vi "Tree.vi"() -> ()   [LabVIEW 2019, in "xy_utilities.lvlib"]
uses:
  xy_utilities.lvlib
  User/User.lvclass
  subVIs/Append (double array).vi
  subVIs/Add float (multiple).vi
  subVIs/Subtract float (multiple).vi
  subVIs/Multiply float (multiple).vi
  subVIs/Divide float (multiple).vi
  subVIs/Add XY (multiple).vi
  subVIs/Subtract XY (multiple).vi
  subVIs/Multiply XY (multiple).vi
  subVIs/Divide XY (multiple).vi
  subVIs/Square Root (multiple).vi
  subVIs/Square (multiple).vi
  subVIs/Reciprocal (multiple).vi
  subVIs/Negate (multiple).vi
  subVIs/Log (multiple).vi
  subVIs/Add float (single).vi
  subVIs/Subtract float (single).vi
  subVIs/Multiply float (single).vi
  subVIs/Divide float (single).vi
  subVIs/Add XY (single).vi
  subVIs/Subtract XY (single).vi
  subVIs/Multiply XY (single).vi
  subVIs/Divide XY (single).vi
  subVIs/Square Root (single).vi
  subVIs/Square (single).vi
  subVIs/Reciprocal (single).vi
  subVIs/Negate (single).vi
  subVIs/Log (single).vi
  <vilib>/Analysis/6fits.llb/Remove Outliers (Range).vi
  <vilib>/Analysis/2dsp.llb/1D Auto Correlation (DBL).vi
  <vilib>/Analysis/2dsp.llb/Decimate (single shot, DBL).vi
  subVIs/Sort (multiple).vi
  subVIs/Reverse (multiple).vi
  subVIs/Decimate (multiple).vi
  subVIs/Subset (multiple).vi
  subVIs/Interpolate Y (multiple).vi
  subVIs/Append (multiple).vi
  subVIs/Split (multiple).vi
  subVIs/Remove Outliers (multiple).vi
  subVIs/Restrict X Range (multiple).vi
  subVIs/Sort (single).vi
  subVIs/Reverse (single).vi
  subVIs/Decimate (single).vi
  subVIs/Subset (single).vi
  subVIs/Interpolate Y (single).vi
  subVIs/Append (double scaler).vi
  subVIs/Append (single).vi
  subVIs/Split (single).vi
  subVIs/Remove Outliers (single).vi
  subVIs/Restrict X Range (single).vi
  subVIs/AutoCorrelation (single).vi
  subVIs/CrossCorrelation (single).vi
  subVIs/Swap X and Y (multiple).vi
  subVIs/Get X and Y (multiple).vi
  subVIs/XY to Waveform (multiple).vi
  subVIs/Get Size (multiple).vi
  subVIs/Max and Min (multiple).vi
  subVIs/Swap X and Y (single).vi
  subVIs/Get X and Y (single).vi
  subVIs/XY to Waveform (single).vi
  subVIs/Get Size (single).vi
  subVIs/Max and Min (single).vi
  <vilib>/Analysis/baseanly.llb/Mean (DBL).vi
  subVIs/Derivative (multiple).vi
  subVIs/Difference Quotient (multiple).vi
  subVIs/Linear Fit (multiple).vi
  subVIs/Interpolate (multiple).vi
  subVIs/Resample (multiple).vi
  subVIs/PS (multiple).vi
  subVIs/FFT (multiple).vi
  subVIs/Symmetrize (multiple).vi
  subVIs/Shift Zero (multiple).vi
  subVIs/Peak Detector (multiple).vi
  subVIs/Derivative (single).vi
  subVIs/Difference Quotient (single).vi
  subVIs/Linear Fit (single).vi
  subVIs/Interpolate (single).vi
  subVIs/Resample (single).vi
  subVIs/PS (single).vi
  subVIs/FFT (single).vi
  subVIs/Symmetrize (single).vi
  subVIs/Shift Zero (single).vi
  subVIs/Peak Detector (single).vi
  <vilib>/Analysis/3filter.llb/Savitzky-Golay Filter (DBL).vi
  subVIs/Zero Phase Lowpass Filter (multiple).vi
  subVIs/Moving Average (multiple).vi
  subVIs/Savitsky Golay Filter (multiple).vi
  subVIs/Savitsky Golay Weighted Filter (multiple).vi
  User/User (multiple).vi
  subVIs/Zero Phase Lowpass Filter (single).vi
  subVIs/Moving Average (single).vi
  subVIs/Savitsky Golay Filter (single).vi
  subVIs/Savitsky Golay Weighted Filter (single).vi
  User/User (single).vi
  subVIs/(x,y) to XY (multiple).vi
  subVIs/XY to (x,y) (multiple).vi
  subVIs/(x,y) to XY (single).vi
  subVIs/XY to (x,y) (single).vi
  subVIs/Waveform to XY (multiple).vi
  subVIs/Waveform to XY (single).vi
  <vilib>/Utility/error.llb/Clear Errors.vi
  Initialize.vi
  <vilib>/Analysis/6fits.llb/Linear Fit Intervals.vi
  <vilib>/Analysis/6fits.llb/Confidence Interval (Linear).vi
  <userlib>/_OpenG.lib/array/array.llb/Sort Array__ogtk.vi
  <userlib>/_OpenG.lib/array/array.llb/Sort 1D Array (DBL)__ogtk.vi
  <userlib>/_OpenG.lib/array/array.llb/Reorder Array2__ogtk.vi
  <userlib>/_OpenG.lib/array/array.llb/Reorder 1D Array2 (DBL)__ogtk.vi
  <vilib>/Utility/error.llb/Error Cluster From Error Code.vi
  <userlib>/_MGI/1D Array/MGI Threshold 1D Array Extended.vi
  <userlib>/_MGI/1D Array/MGI Interpolate 1D Array Extended.vi
  <vilib>/Waveform/WDTOps.llb/WDT Append Waveforms DBL.vi
  <vilib>/Analysis/2dsp.llb/1D Cross Correlation (DBL).vi
  <vilib>/measure/maresamp.llb/Resample Pair of Arrays (single shot).vi
  subVIs/Circular Buffer (waveform).vi
  subVIs/Circular Buffer (single).vi
  subVIs/Circular Buffer (waveforms).vi
  subVIs/Circular Buffer (multiple).vi
  subVIs/Circular Buffer (scaler).vi
  subVIs/Circular Buffer (array).vi
  <vilib>/Analysis/1siggen.llb/Ramp Pattern.vi
  <vilib>/Analysis/1siggen.llb/Ramp Pattern by Delta.vi
  <vilib>/gmath/interp.llb/Interpolate 1D.vi
  <vilib>/measure/maspectr.llb/FFT Power Spectrum and PSD for 1 Chan.vi
  <vilib>/measure/maspectr.llb/FFT Spectrum (Mag-Phase) for 1 Chan.vi
  <vilib>/measure/maresamp.llb/Resample Waveform (single shot).vi
  <vilib>/measure/maresamp.llb/Resample N Pairs of Arrays (single shot).vi
  <vilib>/Analysis/3filter.llb/FIR Windowed Coefficients.vi
  <vilib>/Analysis/3filter.llb/Zero Phase Filter (DBL).vi
  <vilib>/Waveform/WDTOps.llb/Waveform to XY Pairs.vi
  <vilib>/Waveform/WDTOps.llb/WDT Waveform to XY Pairs DBL.vi
  <vilib>/Analysis/NI_AALPro.lvlib
  <vilib>/Analysis/NI_AALBase.lvlib
  <vilib>/measure/NI_MAPro.lvlib
  <vilib>/ptbypt/NI_PtbyPt.lvlib
  <vilib>/Analysis/NI_AAL_SigProc.lvlib
panel:
  out "Array of XY-data":cluster{"X-array":dbl[], "Y-array":dbl[]}[](array[cluster])
  out "XY-data":cluster{"X-array":dbl[], "Y-array":dbl[]}
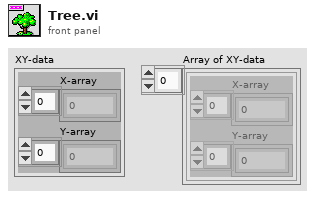
[diagram p1: front panel]
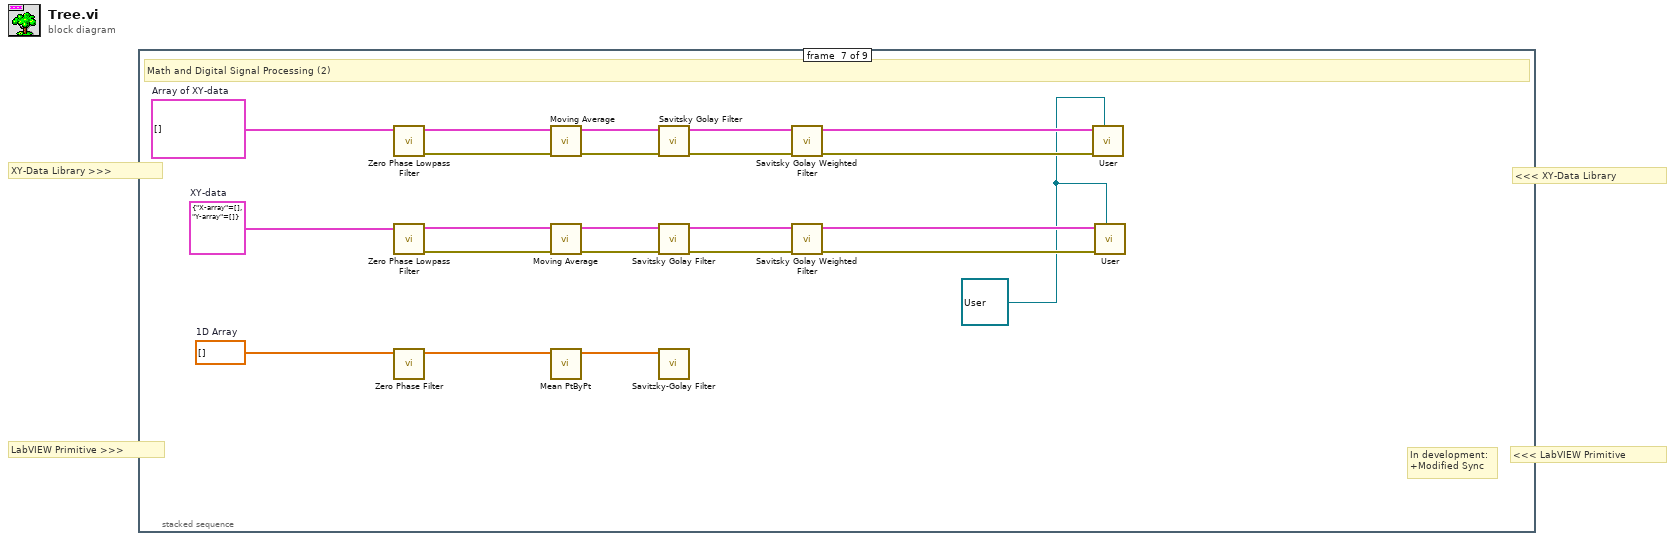
[diagram p0: block diagram]
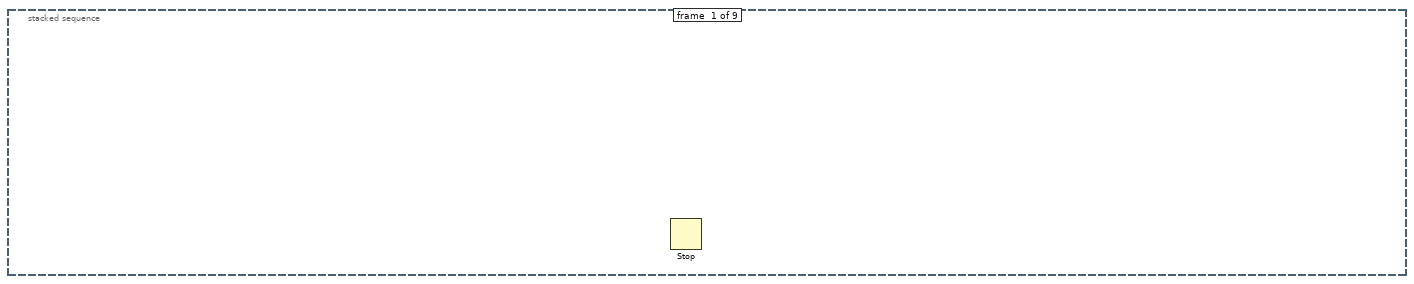
[diagram p2: hidden frame]
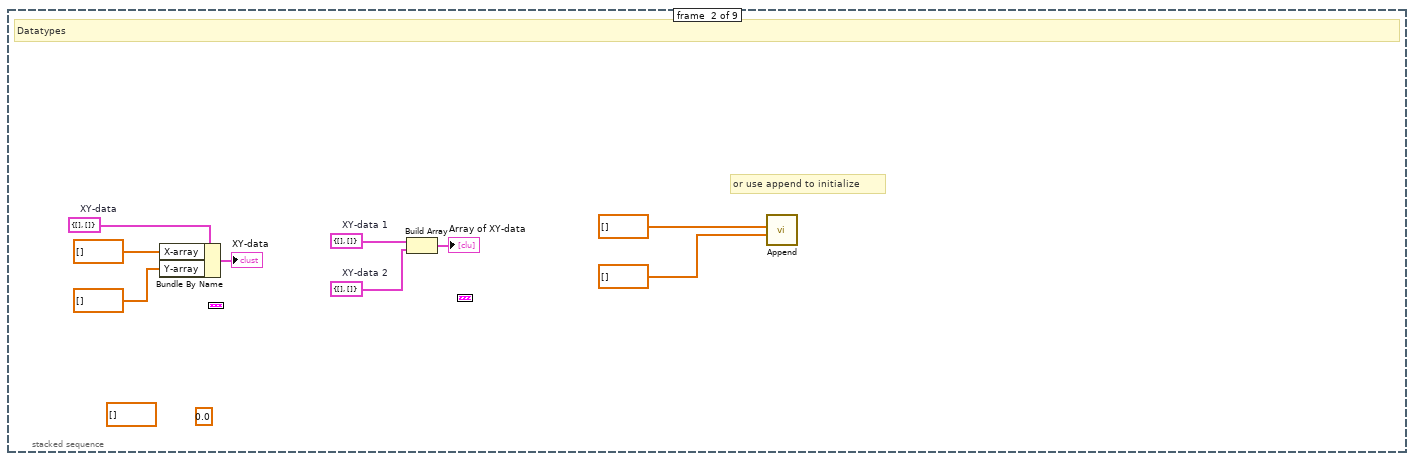
[diagram p3: hidden frame]
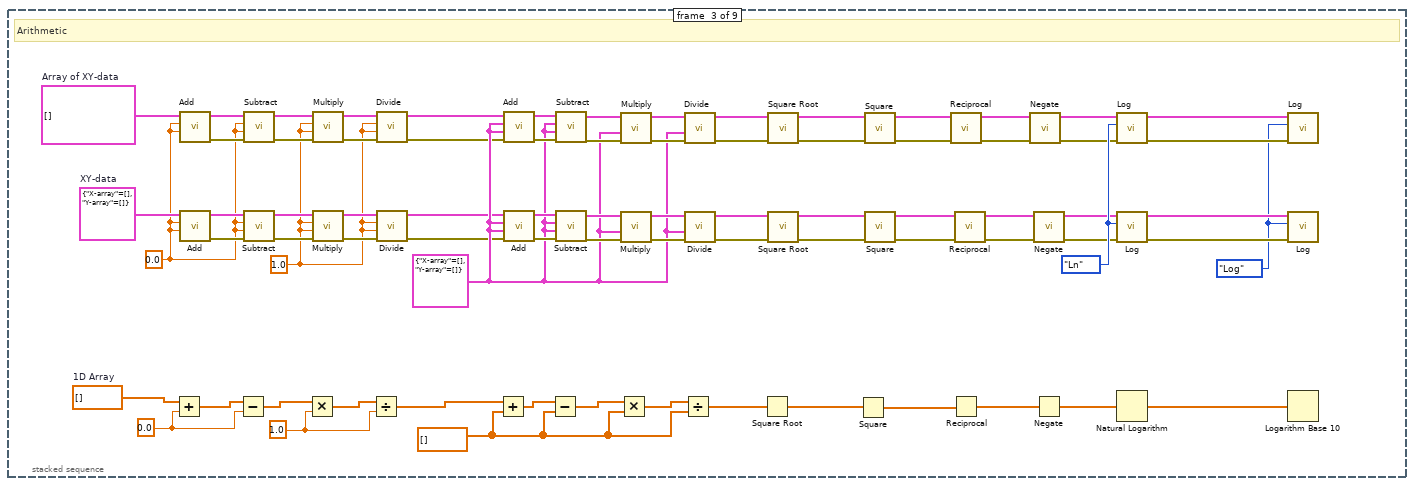
[diagram p4: hidden frame]
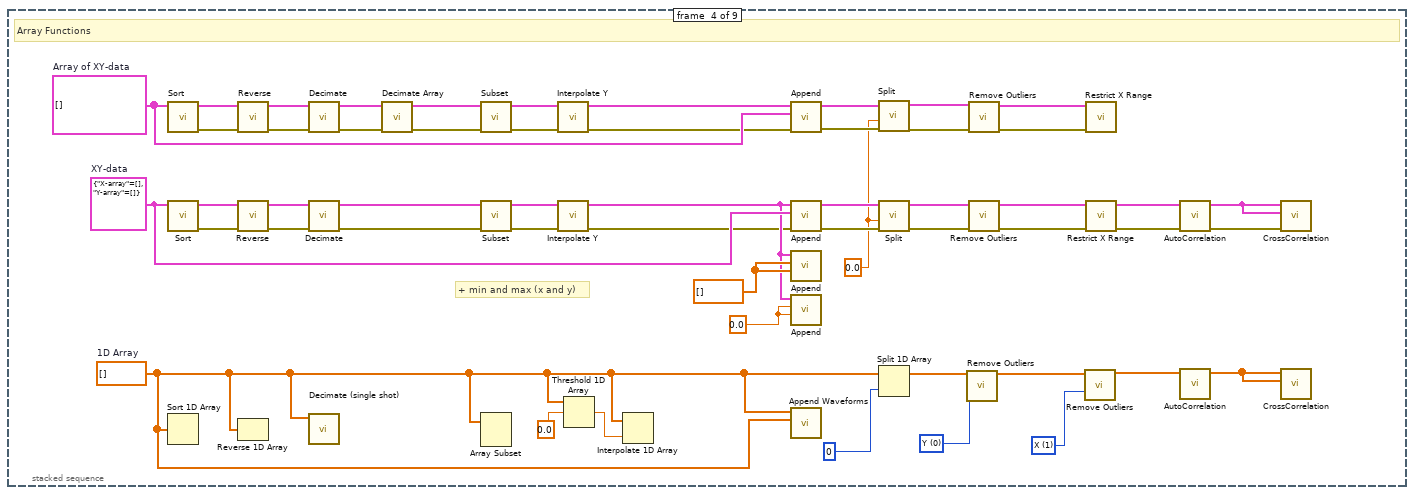
[diagram p5: hidden frame]
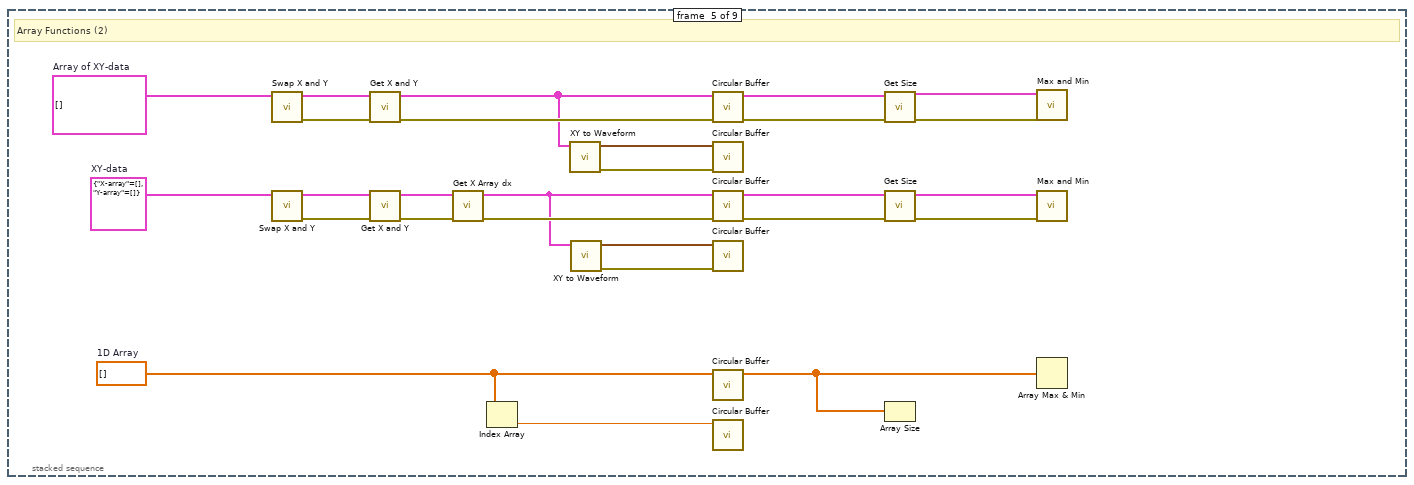
[diagram p6: hidden frame]
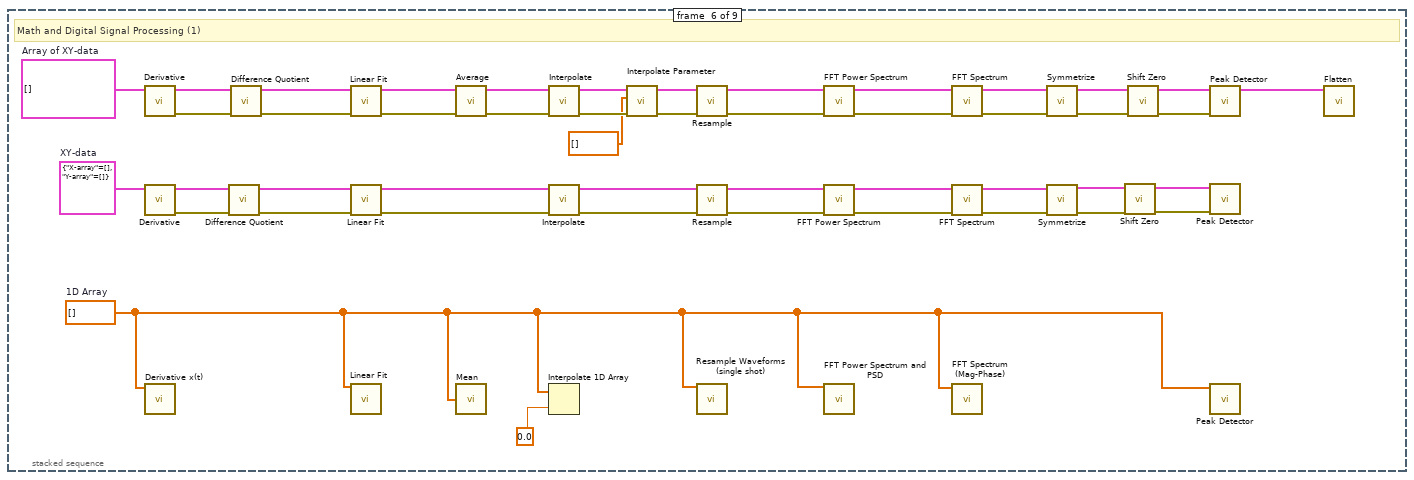
[diagram p7: hidden frame]
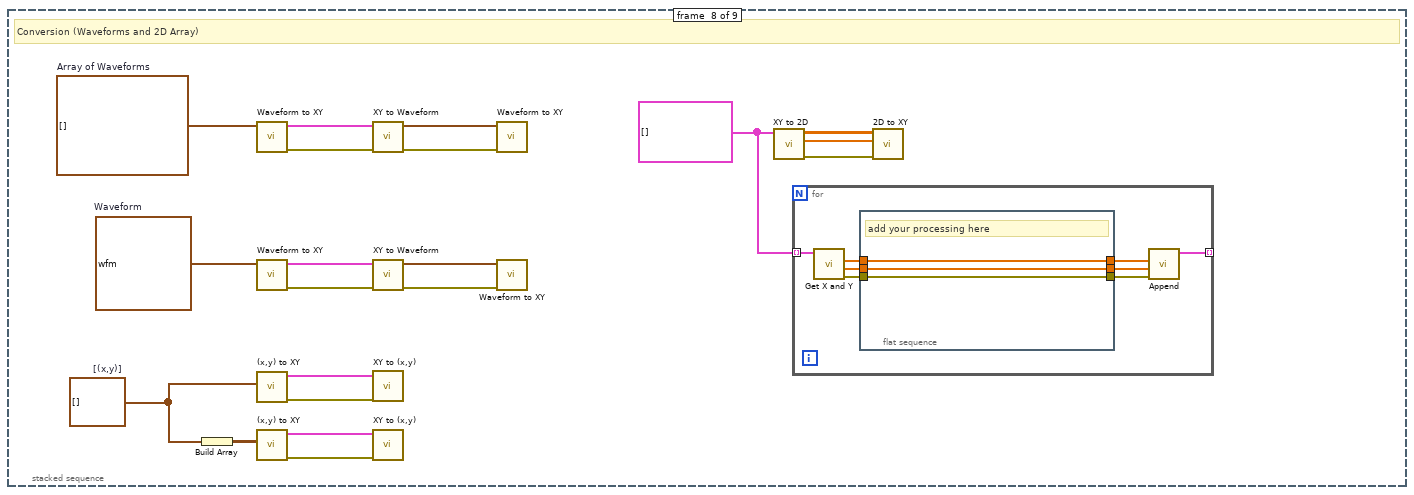
[diagram p8: hidden frame]
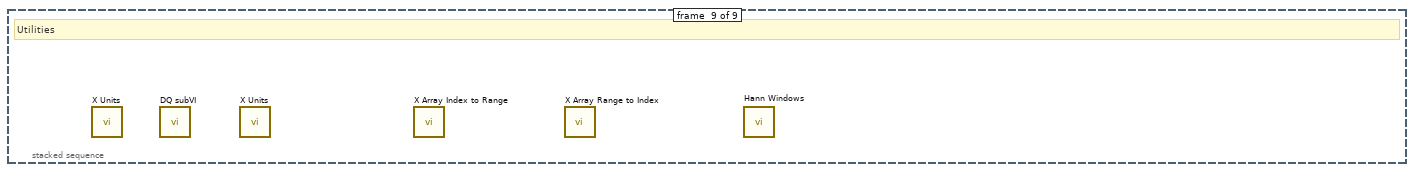
[diagram p9: hidden frame]
diagram:
  # "XY-Data Library >>>"
  # "LabVIEW Primitive >>>"
  # "<<< XY-Data Library"
  # "<<< LabVIEW Primitive"
  n1 = stacked-sequence {
    frame #0 {
      n2 = Stop() -> ()  [unwired: 1 in]
    }
    frame #1 {
      (unwired) 0.0
      (unwired) dbl[] [] ("Y-array")
      w7 = cluster{"X-array":dbl[], "Y-array":dbl[]} {"X-array"=[], "Y-array"=[]}  # XY-data 2
      w8 = cluster{"X-array":dbl[], "Y-array":dbl[]} {"X-array"=[], "Y-array"=[]}  # XY-data 1
      w6 = cluster{"X-array":dbl[], "Y-array":dbl[]} {"X-array"=[], "Y-array"=[]}  # XY-data
      # "or use append to initialize"
      # "Datatypes"
      n3 = Bundle By Name(cluster=w6, "X-array"=dbl[] [], "Y-array"=dbl[] []) -> (→"XY-data":cluster{"X-array":dbl[], "Y-array":dbl[]})
      n4 = Build Array(w8, w7) -> (→"Array of XY-data":cluster{"X-array":dbl[], "Y-array":dbl[]}[])
      n5 = call-poly "Append.vi"("Y-array"=dbl[] [], "X-array"=dbl[] []) -> ()  [unwired: 8 in, 2 out]
    }
    frame #2 {
      w35 = enum16{"Ln", "Log"}."Log" ("Type")
      w41 = enum16{"Ln", "Log"}."Ln" ("Type")
      w51 = cluster{"X-array":dbl[], "Y-array":dbl[]} {"X-array"=[], "Y-array"=[]} ("XY-data in")
      w60 = 1.0 ("x (0)")
      w69 = 0.0 ("x (0)")
      w48 = dbl[] []
      w62 = 1.0 ("x (0)")
      w63 = 0.0 ("x (0)")
      w42 = dbl[] []  # 1D Array
      w85 = cluster{"X-array":dbl[], "Y-array":dbl[]}[] []  # Array of XY-data
      w84 = cluster{"X-array":dbl[], "Y-array":dbl[]} {"X-array"=[], "Y-array"=[]}  # XY-data
      # "Arithmetic"
      n6 = Add(x=w42, y=w63) -> (x+y=w83:dbl[])
      n7 = call-poly "Add.vi"("y (0)"=w69, "x (0)"=w69, "XY-data"=w85) -> ("error out"=w74:errorcluster, "XY-data out"=w75:cluster{"X-array":dbl[], "Y-array":dbl[]}[])  [unwired: 7 in]
      n8 = call-poly "Add.vi"("y (0)"=w69, "x (0)"=w69, "XY-data"=w84) -> ("error out"=w70:errorcluster, "XY-data out"=w71:cluster{"X-array":dbl[], "Y-array":dbl[]})  [unwired: 7 in]
      n9 = Subtract(x=w83, y=w63) -> (x-y=w82:dbl[])
      n10 = call-poly "Subtract.vi"("error in (no error)"=w74, "y (0)"=w69, "x (0)"=w69, "XY-data"=w75) -> ("error out"=w72:errorcluster, "XY-data out"=w73:cluster{"X-array":dbl[], "Y-array":dbl[]}[])  [unwired: 6 in]
      n11 = call-poly "Subtract.vi"("error in (no error)"=w70, "y (0)"=w69, "x (0)"=w69, "XY-data"=w71) -> ("error out"=w77:errorcluster, "XY-data out"=w78:cluster{"X-array":dbl[], "Y-array":dbl[]})  [unwired: 6 in]
      n12 = Multiply(x=w82, y=w62) -> (x*y=w64:dbl[])
      n13 = call-poly "Multiply.vi"("error in (no error)"=w72, "y (1)"=w60, "x (1)"=w60, "XY-data"=w73) -> ("error out"=w79:errorcluster, "XY-data out"=w81:cluster{"X-array":dbl[], "Y-array":dbl[]}[])  [unwired: 6 in]
      n14 = call-poly "Multiply.vi"("error in (no error)"=w77, "y (1)"=w60, "x (1)"=w60, "XY-data"=w78) -> ("error out"=w76:errorcluster, "XY-data out"=w80:cluster{"X-array":dbl[], "Y-array":dbl[]})  [unwired: 6 in]
      n15 = Divide(x=w64, y=w62) -> (x/y=w43:dbl[])
      n16 = call-poly "Divide.vi"("error in (no error)"=w79, "y (1)"=w60, "x (1)"=w60, "XY-data"=w81) -> ("error out"=w46:errorcluster, "XY-data out"=w47:cluster{"X-array":dbl[], "Y-array":dbl[]}[])  [unwired: 6 in]
      n17 = call-poly "Divide.vi"("error in (no error)"=w76, "y (1)"=w60, "x (1)"=w60, "XY-data"=w80) -> ("error out"=w44:errorcluster, "XY-data out"=w45:cluster{"X-array":dbl[], "Y-array":dbl[]})  [unwired: 6 in]
      n18 = Add(x=w43, y=w48) -> (x+y=w61:dbl[])
      n19 = call-poly "Add.vi"("error in (no error)"=w46, "y"=w51, "x"=w51, "XY-data"=w47) -> ("error out"=w67:errorcluster, "XY-data out"=w66:cluster{"X-array":dbl[], "Y-array":dbl[]}[])  [unwired: 6 in]
      n20 = call-poly "Add.vi"("error in (no error)"=w44, "y"=w51, "x"=w51, "XY-data"=w45) -> ("error out"=w65:errorcluster, "XY-data out"=w68:cluster{"X-array":dbl[], "Y-array":dbl[]})  [unwired: 6 in]
      n21 = Subtract(x=w61, y=w48) -> (x-y=w49:dbl[])
      n22 = call-poly "Subtract.vi"("error in (no error)"=w67, "y"=w51, "x"=w51, "XY-data"=w66) -> ("error out"=w54:errorcluster, "XY-data out"=w55:cluster{"X-array":dbl[], "Y-array":dbl[]}[])  [unwired: 6 in]
      n23 = call-poly "Subtract.vi"("error in (no error)"=w65, "y"=w51, "x"=w51, "XY-data"=w68) -> ("error out"=w52:errorcluster, "XY-data out"=w53:cluster{"X-array":dbl[], "Y-array":dbl[]})  [unwired: 6 in]
      n24 = Multiply(x=w49, y=w48) -> (x*y=w50:dbl[])
      n25 = call-poly "Multiply.vi"("error in (no error)"=w54, "y"=w51, "XY-data"=w55) -> ("error out"=w58:errorcluster, "XY-data out"=w56:cluster{"X-array":dbl[], "Y-array":dbl[]}[])  [unwired: 7 in]
      n26 = call-poly "Multiply.vi"("error in (no error)"=w52, "y"=w51, "XY-data"=w53) -> ("error out"=w59:errorcluster, "XY-data out"=w57:cluster{"X-array":dbl[], "Y-array":dbl[]})  [unwired: 7 in]
      n27 = Divide(x=w50, y=w48) -> (x/y=w33:dbl[])
      n28 = call-poly "Divide.vi"("error in (no error)"=w58, "y"=w51, "XY-data"=w56) -> ("error out"=w28:errorcluster, "XY-data out"=w29:cluster{"X-array":dbl[], "Y-array":dbl[]}[])  [unwired: 7 in]
      n29 = call-poly "Divide.vi"("error in (no error)"=w59, "y"=w51, "XY-data"=w57) -> ("error out"=w18:errorcluster, "XY-data out"=w19:cluster{"X-array":dbl[], "Y-array":dbl[]})  [unwired: 7 in]
      n30 = Square Root(x=w33) -> (sqrt(x)=w32:dbl[])
      n31 = call-poly "Square Root.vi"("error in (no error)"=w28, "XY-data"=w29) -> ("error out"=w26:errorcluster, "XY-data out"=w27:cluster{"X-array":dbl[], "Y-array":dbl[]}[])  [unwired: 8 in]
      n32 = call-poly "Square Root.vi"("error in (no error)"=w18, "XY-data"=w19) -> ("error out"=w16:errorcluster, "XY-data out"=w17:cluster{"X-array":dbl[], "Y-array":dbl[]})  [unwired: 8 in]
      n33 = Square(x=w32) -> (x^2=w31:dbl[])
      n34 = call-poly "Square.vi"("error in (no error)"=w26, "XY-data"=w27) -> ("error out"=w24:errorcluster, "XY-data out"=w25:cluster{"X-array":dbl[], "Y-array":dbl[]}[])  [unwired: 8 in]
      n35 = call-poly "Square.vi"("error in (no error)"=w16, "XY-data"=w17) -> ("error out"=w14:errorcluster, "XY-data out"=w15:cluster{"X-array":dbl[], "Y-array":dbl[]})  [unwired: 8 in]
      n36 = call-poly "Reciprocal.vi"("error in (no error)"=w24, "XY-data"=w25) -> ("error out"=w22:errorcluster, "XY-data out"=w23:cluster{"X-array":dbl[], "Y-array":dbl[]}[])  [unwired: 8 in]
      n37 = Reciprocal(x=w31) -> (1/x=w36:dbl[])
      n38 = call-poly "Reciprocal.vi"("error in (no error)"=w14, "XY-data"=w15) -> ("error out"=w12:errorcluster, "XY-data out"=w13:cluster{"X-array":dbl[], "Y-array":dbl[]})  [unwired: 8 in]
      n39 = call-poly "Negate.vi"("error in (no error)"=w22, "XY-data"=w23) -> ("error out"=w20:errorcluster, "XY-data out"=w21:cluster{"X-array":dbl[], "Y-array":dbl[]}[])  [unwired: 8 in]
      n40 = call-poly "Negate.vi"("error in (no error)"=w12, "XY-data"=w13) -> ("error out"=w10:errorcluster, "XY-data out"=w11:cluster{"X-array":dbl[], "Y-array":dbl[]})  [unwired: 8 in]
      n41 = Negate(x=w36) -> (-x=w30:dbl[])
      n42 = call-poly "Log.vi"("error in (no error)"=w20, "Type"=w41, "XY-data"=w21) -> ("error out"=w39:errorcluster, "XY-data out"=w40:cluster{"X-array":dbl[], "Y-array":dbl[]}[])  [unwired: 7 in]
      n43 = call-poly "Log.vi"("error in (no error)"=w10, "Type"=w41, "XY-data"=w11) -> ("error out"=w37:errorcluster, "XY-data out"=w38:cluster{"X-array":dbl[], "Y-array":dbl[]})  [unwired: 7 in]
      n44 = Natural Logarithm(1:w30) -> (0:w34:dbl[])
      n45 = call-poly "Log.vi"("error in (no error)"=w39, "Type"=w35, "XY-data"=w40) -> ()  [unwired: 7 in, 2 out]
      n46 = call-poly "Log.vi"("error in (no error)"=w37, "Type"=w35, "XY-data"=w38) -> ()  [unwired: 7 in, 2 out]
      n47 = Logarithm Base 10(1:w34) -> ()  [unwired: 1 out]
    }
    frame #3 {
      w92 = 0.0 ("index")
      w112 = dbl[] [] ("1D Array")
      w113 = u16 1 items=["Y", "X", "X and Y"] ("range type")
      w114 = u16 0 items=["Y", "X", "X and Y"] ("range type")
      w111 = 0.0 ("threshold y")
      w98 = dbl[] []  # 1D Array
      w109 = cluster{"X-array":dbl[], "Y-array":dbl[]}[] []  # Array of XY-data
      w110 = cluster{"X-array":dbl[], "Y-array":dbl[]} {"X-array"=[], "Y-array"=[]}  # XY-data
      # "+ min and max (x and y)"
      # "Array Functions"
      n48 = call-poly "Sort.vi"("XY-data"=w109) -> ("error out"=w133:errorcluster, "Sorted XY-data out"=w134:cluster{"X-array":dbl[], "Y-array":dbl[]}[])  [unwired: 8 in, 1 out]
      n49 = call-poly "Sort.vi"("XY-data"=w110) -> ("error out"=w129:errorcluster, "Sorted XY-data out"=w130:cluster{"X-array":dbl[], "Y-array":dbl[]})  [unwired: 8 in, 1 out]
      n50 = Sort 1D Array(array=w98) -> ()  [unwired: 1 out]
      n51 = call-poly "Reverse.vi"("error in (no error)"=w133, "XY-data"=w134) -> ("error out"=w131:errorcluster, "Reversed XY-data out"=w132:cluster{"X-array":dbl[], "Y-array":dbl[]}[])  [unwired: 8 in]
      n52 = call-poly "Reverse.vi"("error in (no error)"=w129, "XY-data"=w130) -> ("error out"=w136:errorcluster, "Reversed XY-data out"=w135:cluster{"X-array":dbl[], "Y-array":dbl[]})  [unwired: 8 in]
      n53 = Reverse 1D Array(array=w98) -> ()  [unwired: 1 out]
      n54 = call-poly "Decimate.vi"("error in (no error)"=w131, "XY-data"=w132) -> ("error out"=w128:errorcluster, "Decimated XY-data out"=w127:cluster{"X-array":dbl[], "Y-array":dbl[]}[])  [unwired: 8 in]
      n55 = call-poly "Decimate.vi"("error in (no error)"=w136, "XY-data"=w135) -> ("error out"=w137:errorcluster, "Decimated XY-data out"=w138:cluster{"X-array":dbl[], "Y-array":dbl[]})  [unwired: 8 in]
      n56 = call-poly <vilib>:"Decimate (single shot).vi"("X"=w98) -> ()  [unwired: 9 in, 2 out]
      n57 = call "Decimate Array.vi"("error in (no error)"=w128, "XY-data"=w127) -> ("error out"=w126:errorcluster, "Decimated XY-data out"=w125:cluster{"X-array":dbl[], "Y-array":dbl[]}[])  [unwired: 8 in]
      n58 = call-poly "Subset.vi"("error in (no error)"=w126, "XY-data"=w125) -> ("error out"=w123:errorcluster, "Subset XY-data out"=w124:cluster{"X-array":dbl[], "Y-array":dbl[]}[])  [unwired: 8 in]
      n59 = call-poly "Subset.vi"("error in (no error)"=w137, "XY-data"=w138) -> ("error out"=w121:errorcluster, "XY-data out"=w122:cluster{"X-array":dbl[], "Y-array":dbl[]})  [unwired: 8 in]
      n60 = Array Subset "Array Subset"(array=w98) -> ()  [unwired: 2 in, 1 out]
      n61 = call-poly "Interpolate Y.vi"("error in (no error)"=w123, "XY-data"=w124) -> ("error out"=w106:errorcluster, "XY-data out"=w107:cluster{"X-array":dbl[], "Y-array":dbl[]}[])  [unwired: 7 in, 1 out]
      n62 = call-poly "Interpolate Y.vi"("error in (no error)"=w121, "XY-data"=w122) -> ("error out"=w104:errorcluster, "XY-data out"=w105:cluster{"X-array":dbl[], "Y-array":dbl[]})  [unwired: 7 in, 1 out]
      n63 = Threshold 1D Array(2:0.0 ("threshold y"), 3:w98) -> (0:w120:dbl)  [unwired: 1 in]
      n64 = Interpolate 1D Array(1:w120, 2:w98) -> ()  [unwired: 1 out]
      n65 = call-poly "Append.vi"("error in (no error)"=w106, "XY-data (B)"=w109, "XY-data (A)"=w107) -> ("error out"=w102:errorcluster, "XY-data out"=w103:cluster{"X-array":dbl[], "Y-array":dbl[]}[])  [unwired: 7 in]
      n66 = call-poly "Append.vi"("error in (no error)"=w104, "XY-data (B)"=w110, "XY-data (A)"=w105) -> ("error out"=w95:errorcluster, "XY-data out"=w100:cluster{"X-array":dbl[], "Y-array":dbl[]})  [unwired: 7 in]
      n67 = call-poly "Append.vi"("Y-array"=w112, "X-array"=w112, "XY-data (A)"=w105) -> ()  [unwired: 7 in, 2 out]
      n68 = call-poly "Append.vi"("Y"=w111, "X"=w111, "XY-data (A)"=w105) -> ()  [unwired: 7 in, 2 out]
      n69 = call-poly <vilib>:"Append Waveforms.vi"("waveform B"=w98, "waveform A"=w98) -> ()  [unwired: 8 in, 2 out]
      n70 = call-poly "Split.vi"("error in (no error)"=w102, "fractional index"=w92, "XY-data"=w103) -> ("error out"=w96:errorcluster, "XY-data (A) out"=w101:cluster{"X-array":dbl[], "Y-array":dbl[]}[])  [unwired: 6 in, 1 out]
      n71 = call-poly "Split.vi"("error in (no error)"=w95, "fractional index"=w92, "XY-data"=w100) -> ("error out"=w94:errorcluster, "XY-data (A) out"=w99:cluster{"X-array":dbl[], "Y-array":dbl[]})  [unwired: 6 in, 1 out]
      n72 = Split 1D Array(array=w98, index=0) -> (first subarray=w97:dbl[])  [unwired: 1 out]
      n73 = call-poly <vilib>:"Remove Outliers.vi"("Y"=w97, "range type"=w114) -> ("Y Out"=w115:dbl[])  [unwired: 9 in, 4 out]
      n74 = call-poly <vilib>:"Remove Outliers.vi"("error in (no error)"=w96, "XY-data"=w101) -> ("error out"=w118:errorcluster, "XY-data out"=w119:cluster{"X-array":dbl[], "Y-array":dbl[]}[])  [unwired: 8 in]
      n75 = call-poly <vilib>:"Remove Outliers.vi"("error in (no error)"=w94, "XY-data"=w99) -> ("error out"=w117:errorcluster, "XY-data out"=w116:cluster{"X-array":dbl[], "Y-array":dbl[]})  [unwired: 8 in]
      n76 = call-poly <vilib>:"Remove Outliers.vi"("Y"=w115, "range type"=w113) -> ("Y Out"=w87:dbl[])  [unwired: 9 in, 4 out]
      n77 = call-poly "Restrict X Range.vi"("error in (no error)"=w118, "XY-data"=w119) -> ()  [unwired: 8 in, 2 out]
      n78 = call-poly "Restrict X Range.vi"("error in (no error)"=w117, "XY-data"=w116) -> ("error out"=w90:errorcluster, "XY-data out"=w91:cluster{"X-array":dbl[], "Y-array":dbl[]})  [unwired: 8 in]
      n79 = call-poly <vilib>:"AutoCorrelation.vi"("error in (no error)"=w90, "XY-data a"=w91) -> ("error out"=w89:errorcluster, "XY-data a out"=w88:cluster{"X-array":dbl[], "Y-array":dbl[]})  [unwired: 8 in]
      n80 = call-poly <vilib>:"AutoCorrelation.vi"("X"=w87) -> ("Rxx"=w86:dbl[])  [unwired: 9 in, 1 out]
      n81 = call-poly <vilib>:"CrossCorrelation.vi"("error in (no error)"=w89, "XY-data b"=w88, "XY-data a"=w88) -> ()  [unwired: 6 in, 3 out]
      n82 = call-poly <vilib>:"CrossCorrelation.vi"("Y"=w86, "X"=w86) -> ()  [unwired: 8 in, 2 out]
    }
    frame #4 {
      w151 = dbl[] []  # 1D Array
      w162 = cluster{"X-array":dbl[], "Y-array":dbl[]}[] []  # Array of XY-data
      w160 = cluster{"X-array":dbl[], "Y-array":dbl[]} {"X-array"=[], "Y-array"=[]}  # XY-data
      # "Array Functions (2)"
      n83 = call-poly "Swap X and Y.vi"("XY-data"=w162) -> ("error out"=w165:errorcluster, "XY-data out"=w161:cluster{"X-array":dbl[], "Y-array":dbl[]}[])  [unwired: 9 in]
      n84 = call-poly "Swap X and Y.vi"("XY-data"=w160) -> ("error out"=w163:errorcluster, "XY-data out"=w164:cluster{"X-array":dbl[], "Y-array":dbl[]})  [unwired: 9 in]
      n85 = call-poly "Get X and Y.vi"("error in (no error)"=w165, "XY-data"=w161) -> ("error out"=w158:errorcluster, "XY-data out"=w149:cluster{"X-array":dbl[], "Y-array":dbl[]}[])  [unwired: 6 in, 2 out]
      n86 = call-poly "Get X and Y.vi"("error in (no error)"=w163, "XY-data"=w164) -> ("error out"=w156:errorcluster, "XY-data out"=w159:cluster{"X-array":dbl[], "Y-array":dbl[]})  [unwired: 6 in, 2 out]
      n87 = call "Get X Array dx.vi"("error in (no error)"=w156, "XY-data"=w159) -> ("error out"=w157:errorcluster, "XY-data out"=w148:cluster{"X-array":dbl[], "Y-array":dbl[]})  [unwired: 6 in, 2 out]
      n88 = Index Array(array=w151) -> (element=w150:dbl)  [unwired: 1 in]
      n89 = call-poly "XY to Waveform.vi"("XY-data in"=w149) -> ("error out"=w145:errorcluster, "Waveform out"=w146:waveform(dbl)[])  [unwired: 8 in, 1 out]
      n90 = call-poly "XY to Waveform.vi"("XY-data in"=w148) -> ("error out"=w144:errorcluster, "Waveform out"=w147:waveform(dbl))  [unwired: 8 in, 1 out]
      n91 = call-poly "Circular Buffer.vi"("error in"=w158, "XY-data"=w149) -> ("error out"=w152:errorcluster, "XY-data out"=w154:cluster{"X-array":dbl[], "Y-array":dbl[]}[])  [unwired: 8 in]
      n92 = call-poly "Circular Buffer.vi"("error in"=w145, "Waveform in"=w146) -> ()  [unwired: 8 in, 2 out]
      n93 = call-poly "Circular Buffer.vi"("error in"=w157, "XY-data"=w148) -> ("error out"=w153:errorcluster, "XY-data out"=w155:cluster{"X-array":dbl[], "Y-array":dbl[]})  [unwired: 8 in]
      n94 = call-poly "Circular Buffer.vi"("error in"=w144, "Waveform in"=w147) -> ()  [unwired: 8 in, 2 out]
      n95 = call-poly "Circular Buffer.vi"("Array in"=w151) -> ("Array out"=w139:dbl[])  [unwired: 9 in, 1 out]
      n96 = call-poly "Circular Buffer.vi"("Element in"=w150) -> ()  [unwired: 9 in, 2 out]
      n97 = call-poly "Get Size.vi"("error in (no error)"=w152, "XY-data"=w154) -> ("error out"=w143:errorcluster, "XY-data out"=w142:cluster{"X-array":dbl[], "Y-array":dbl[]}[])  [unwired: 6 in, 2 out]
      n98 = call-poly "Get Size.vi"("error in (no error)"=w153, "XY-data"=w155) -> ("error out"=w140:errorcluster, "XY-data out"=w141:cluster{"X-array":dbl[], "Y-array":dbl[]})  [unwired: 6 in, 2 out]
      n99 = Array Size(array=w139) -> ()  [unwired: 1 out]
      n100 = call-poly "Max and Min.vi"("error in (no error)"=w143, "XY-data"=w142) -> ()  [unwired: 6 in, 4 out]
      n101 = call-poly "Max and Min.vi"("error in (no error)"=w140, "XY-data"=w141) -> ()  [unwired: 6 in, 4 out]
      n102 = Array Max & Min(array=w139) -> ()  [unwired: 4 out]
    }
    frame #5 {
      w169 = dbl[] []  # 1D Array
      w200 = cluster{"X-array":dbl[], "Y-array":dbl[]}[] []  # Array of XY-data
      w199 = cluster{"X-array":dbl[], "Y-array":dbl[]} {"X-array"=[], "Y-array"=[]}  # XY-data
      # "Math and Digital Signal Processing (1)"
      n103 = call-poly "Derivative.vi"("XY-data"=w200) -> ("error out"=w182:errorcluster, "XY-data out"=w183:cluster{"X-array":dbl[], "Y-array":dbl[]}[])  [unwired: 8 in, 1 out]
      n104 = call-poly "Derivative.vi"("XY-data"=w199) -> ("error out"=w172:errorcluster, "XY-data out"=w176:cluster{"X-array":dbl[], "Y-array":dbl[]})  [unwired: 8 in, 1 out]
      n105 = call <vilib>:"Derivative x(t).vi"("X"=w169) -> ()  [unwired: 9 in, 2 out]
      n106 = call-poly "Difference Quotient.vi"("error in (no error)"=w172, "XY-data"=w176) -> ("error out"=w177:errorcluster, "XY-data out"=w175:cluster{"X-array":dbl[], "Y-array":dbl[]})  [unwired: 7 in, 1 out]
      n107 = call-poly "Difference Quotient.vi"("error in (no error)"=w182, "XY-data"=w183) -> ("error out"=w180:errorcluster, "XY-data out"=w181:cluster{"X-array":dbl[], "Y-array":dbl[]}[])  [unwired: 7 in, 1 out]
      n108 = call-poly <vilib>:"Linear Fit.vi"("error in (no error)"=w180, "XY-data"=w181) -> ("error out"=w179:errorcluster, "XY-data out"=w178:cluster{"X-array":dbl[], "Y-array":dbl[]}[])  [unwired: 3 in, 5 out]
      n109 = call-poly <vilib>:"Linear Fit.vi"("error in (no error)"=w177, "XY-data"=w175) -> ("error out"=w173:errorcluster, "XY-data out"=w174:cluster{"X-array":dbl[], "Y-array":dbl[]})  [unwired: 3 in, 5 out]
      n110 = call <vilib>:"Linear Fit.vi"("Y"=w169) -> ()  [unwired: 10 in, 5 out]
      n111 = call "Average.vi"("error in (no error)"=w179, "XY-data"=w178) -> ("error out"=w205:errorcluster, "XY-data out"=w206:cluster{"X-array":dbl[], "Y-array":dbl[]}[])  [unwired: 7 in, 1 out]
      n112 = call-poly <vilib>:"Mean.vi"("X"=w169) -> ()  [unwired: 2 out]
      n113 = call-poly "Interpolate.vi"("error in (no error)"=w205, "XY-data"=w206) -> ("error out"=w187:errorcluster, "Interpolated XY-data out"=w189:cluster{"X-array":dbl[], "Y-array":dbl[]}[])  [unwired: 8 in]
      n114 = call-poly "Interpolate.vi"("error in (no error)"=w173, "XY-data"=w174) -> ("error out"=w207:errorcluster, "Interpolated XY-data out"=w190:cluster{"X-array":dbl[], "Y-array":dbl[]})  [unwired: 8 in]
      n115 = Interpolate 1D Array(1:0.0 ("fractional index or x"), 2:w169) -> ()  [unwired: 1 out]
      n116 = call "Interpolate Parameter.vi"("error in (no error)"=w187, "Parameter-array"=dbl[] [] ("1D Array"), "XY-data"=w189) -> ("error out"=w186:errorcluster, "Interpolated XY-data out"=w188:cluster{"X-array":dbl[], "Y-array":dbl[]}[])  [unwired: 6 in, 1 out]
      n117 = call-poly "Resample.vi"("error in (no error)"=w186, "XY-data"=w188) -> ("error out"=w203:errorcluster, "Resampled XY-data out"=w204:cluster{"X-array":dbl[], "Y-array":dbl[]}[])  [unwired: 8 in]
      n118 = call-poly "Resample.vi"("error in (no error)"=w207, "XY-data"=w190) -> ("error out"=w201:errorcluster, "Resampled XY-data out"=w202:cluster{"X-array":dbl[], "Y-array":dbl[]})  [unwired: 8 in]
      n119 = call-poly <vilib>:"Resample Waveforms (single shot).vi"("waveform in"=w169) -> ()  [unwired: 11 in, 4 out]
      n120 = call-poly "FFT Power Spectrum.vi"("error in (no error)"=w203, "XY-data"=w204) -> ("error out"=w209:errorcluster, "XY-data out"=w210:cluster{"X-array":dbl[], "Y-array":dbl[]}[])  [unwired: 7 in, 1 out]
      n121 = call-poly "FFT Power Spectrum.vi"("error in (no error)"=w201, "XY-data"=w202) -> ("error out"=w208:errorcluster, "XY-data out"=w211:cluster{"X-array":dbl[], "Y-array":dbl[]})  [unwired: 7 in, 1 out]
      n122 = call-poly <vilib>:"FFT Power Spectrum and PSD.vi"("time signal"=w169) -> ()  [unwired: 7 in, 4 out]
      n123 = call-poly "FFT Spectrum.vi"("error in (no error)"=w209, "XY-data"=w210) -> ("error out"=w195:errorcluster, "XY-data out"=w198:cluster{"X-array":dbl[], "Y-array":dbl[]}[])  [unwired: 6 in, 2 out]
      n124 = call-poly "FFT Spectrum.vi"("error in (no error)"=w208, "XY-data"=w211) -> ("error out"=w196:errorcluster, "XY-data out"=w197:cluster{"X-array":dbl[], "Y-array":dbl[]})  [unwired: 6 in, 2 out]
      n125 = call-poly <vilib>:"FFT Spectrum (Mag-Phase).vi"("time signal"=w169) -> ()  [unwired: 6 in, 5 out]
      n126 = call-poly "Symmetrize.vi"("error in (no error)"=w195, "XY-data"=w198) -> ("error out"=w192:errorcluster, "XY-data out"=w191:cluster{"X-array":dbl[], "Y-array":dbl[]}[])  [unwired: 6 in, 2 out]
      n127 = call-poly "Symmetrize.vi"("error in (no error)"=w196, "XY-data"=w197) -> ("error out"=w194:errorcluster, "XY-data out"=w193:cluster{"X-array":dbl[], "Y-array":dbl[]})  [unwired: 6 in, 2 out]
      n128 = call-poly "Shift Zero.vi"("error in (no error)"=w194, "XY-data"=w193) -> ("error out"=w168:errorcluster, "Shifted XY-data out"=w171:cluster{"X-array":dbl[], "Y-array":dbl[]})  [unwired: 8 in]
      n129 = call-poly "Shift Zero.vi"("error in (no error)"=w192, "XY-data"=w191) -> ("error out"=w167:errorcluster, "Shifted XY-data out"=w170:cluster{"X-array":dbl[], "Y-array":dbl[]}[])  [unwired: 8 in]
      n130 = call-poly <vilib>:"Peak Detector.vi"("error in (no error)"=w167, "XY-data"=w170) -> ("XY-data out"=w166:cluster{"X-array":dbl[], "Y-array":dbl[]}[])  [unwired: 6 in, 3 out]
      n131 = call-poly <vilib>:"Peak Detector.vi"("error in (no error)"=w168, "XY-data"=w171) -> ()  [unwired: 6 in, 4 out]
      n132 = call <vilib>:"Peak Detector.vi"("X"=w169) -> ()  [unwired: 6 in, 5 out]
      n133 = call "Flatten.vi"("XY-data"=w166) -> ()  [unwired: 9 in, 2 out]
    }
    frame #6 {
      w212 = refnum<class "User.lvclass"> refnum ("User.lvclass")
      w222 = dbl[] []  # 1D Array
      w231 = cluster{"X-array":dbl[], "Y-array":dbl[]}[] []  # Array of XY-data
      w232 = cluster{"X-array":dbl[], "Y-array":dbl[]} {"X-array"=[], "Y-array"=[]}  # XY-data
      # "In development:\n+Modified Sync"
      # "Math and Digital Signal Processing (2)"
      n134 = call-poly "Zero Phase Lowpass Filter.vi"("XY-data"=w231) -> ("error out"=w229:errorcluster, "XY-data out"=w230:cluster{"X-array":dbl[], "Y-array":dbl[]}[])  [unwired: 9 in]
      n135 = call-poly "Zero Phase Lowpass Filter.vi"("XY-data"=w232) -> ("error out"=w228:errorcluster, "XY-data out"=w227:cluster{"X-array":dbl[], "Y-array":dbl[]})  [unwired: 9 in]
      n136 = call-poly <vilib>:"Zero Phase Filter.vi"("X"=w222) -> ("Filtered X"=w221:dbl[])  [unwired: 9 in, 1 out]
      n137 = call-poly "Moving Average.vi"("error in (no error)"=w229, "XY-data"=w230) -> ("error out"=w225:errorcluster, "XY-data out"=w226:cluster{"X-array":dbl[], "Y-array":dbl[]}[])  [unwired: 8 in]
      n138 = call-poly "Moving Average.vi"("error in (no error)"=w228, "XY-data"=w227) -> ("error out"=w224:errorcluster, "XY-data out"=w223:cluster{"X-array":dbl[], "Y-array":dbl[]})  [unwired: 8 in]
      n139 = call <vilib>:"Mean PtByPt.vi"() -> ()  [unwired: 4 in, 2 out]
      n140 = call-poly "Savitsky Golay Filter.vi"("error in (no error)"=w225, "XY-data"=w226) -> ("error out"=w216:errorcluster, "XY-data out"=w220:cluster{"X-array":dbl[], "Y-array":dbl[]}[])  [unwired: 8 in]
      n141 = call-poly "Savitsky Golay Filter.vi"("error in (no error)"=w224, "XY-data"=w223) -> ("error out"=w215:errorcluster, "XY-data out"=w219:cluster{"X-array":dbl[], "Y-array":dbl[]})  [unwired: 8 in]
      n142 = call-poly <vilib>:"Savitzky-Golay Filter.vi"("X"=w221) -> ()  [unwired: 9 in, 2 out]
      n143 = call-poly "Savitsky Golay Weighted Filter.vi"("error in (no error)"=w216, "XY-data"=w220) -> ("error out"=w214:errorcluster, "XY-data out"=w218:cluster{"X-array":dbl[], "Y-array":dbl[]}[])  [unwired: 8 in]
      n144 = call-poly "Savitsky Golay Weighted Filter.vi"("error in (no error)"=w215, "XY-data"=w219) -> ("error out"=w213:errorcluster, "XY-data out"=w217:cluster{"X-array":dbl[], "Y-array":dbl[]})  [unwired: 8 in]
      n145 = call-poly "User.vi"("User.lvclass"=w212, "error in (no error)"=w214, "XY-data"=w218) -> ()  [unwired: 6 in, 3 out]
      n146 = call-poly "User.vi"("User.lvclass"=w212, "error in (no error)"=w213, "XY-data"=w217) -> ()  [unwired: 6 in, 3 out]
    }
    frame #7 {
      w236 = cluster{"x":dbl, "y":dbl}[] []  # [(x,y)]
      w239 = cluster{"X-array":dbl[], "Y-array":dbl[]}[] [] ("XY-data")
      w251 = waveform(dbl)[] []  # Array of Waveforms
      w252 = waveform(dbl) {"t0"=timestamp(0 s since 1904-01-01), "dt"=1.0, "Y"=[]}  # Waveform
      # "Conversion (Waveforms and 2D Array)"
      n147 = Build Array(w236) -> (w235:cluster{"x":dbl, "y":dbl}[][])
      n148 = call-poly "Waveform to XY.vi"("Waveform in"=w251) -> ("error out"=w249:errorcluster, "XY-data out"=w243:cluster{"X-array":dbl[], "Y-array":dbl[]}[])  [unwired: 9 in]
      n149 = call-poly "Waveform to XY.vi"("Waveform in"=w252) -> ("error out"=w245:errorcluster, "XY-data out"=w250:cluster{"X-array":dbl[], "Y-array":dbl[]})  [unwired: 9 in]
      n150 = call-poly "(x,y) to XY.vi"("[(x,y)]"=w236) -> ("error out"=w238:errorcluster, "XY-data out"=w237:cluster{"X-array":dbl[], "Y-array":dbl[]})  [unwired: 9 in]
      n151 = call-poly "(x,y) to XY.vi"("[[(x,y)]]"=w235) -> ("error out"=w233:errorcluster, "XY-data out"=w234:cluster{"X-array":dbl[], "Y-array":dbl[]}[])  [unwired: 9 in]
      n152 = call-poly "XY to Waveform.vi"("error in (no error)"=w249, "XY-data in"=w243) -> ("error out"=w246:errorcluster, "Waveform out"=w248:waveform(dbl)[])  [unwired: 7 in, 1 out]
      n153 = call-poly "XY to Waveform.vi"("error in (no error)"=w245, "XY-data in"=w250) -> ("error out"=w244:errorcluster, "Waveform out"=w247:waveform(dbl))  [unwired: 7 in, 1 out]
      n154 = call-poly "XY to (x,y).vi"("error in (no error)"=w238, "XY-data"=w237) -> ()  [unwired: 7 in, 3 out]
      n155 = call-poly "XY to (x,y).vi"("error in (no error)"=w233, "XY-data"=w234) -> ()  [unwired: 7 in, 3 out]
      n156 = call-poly "Waveform to XY.vi"("error in (no error)"=w246, "Waveform in"=w248) -> ()  [unwired: 8 in, 2 out]
      n157 = call-poly "Waveform to XY.vi"("error in (no error)"=w244, "Waveform in"=w247) -> ()  [unwired: 8 in, 2 out]
      n158 = call "XY to 2D.vi"("XY-data"=w239) -> ("error out"=w240:errorcluster, "X Array"=w241:dbl[], "2D Z Array"=w242:dbl[][])  [unwired: 7 in, 1 out]
      n159 = for {
        tunnel: w239 -> [w260] mode=indexing
        tunnel: [w259] -> _ mode=indexing
        n160 = call-poly "Get X and Y.vi"("XY-data"=w260) -> ("error out"=w257:errorcluster, "Y-array"=w255:dbl[], "X-array"=w258:dbl[])  [unwired: 7 in, 1 out]
        n161 = flat-sequence {
          tunnel: w258 -> [w261]
          tunnel: w257 -> [w262]
          tunnel: [w263] -> w256
          tunnel: w255 -> [w263]
          tunnel: [w262] -> w254
          tunnel: [w261] -> w253
          frame #0 {
            # "add your processing here"
          }
        }
        n162 = call-poly "Append.vi"("error in (no error)"=w254, "Y-array"=w256, "X-array"=w253) -> ("XY-data out"=w259:cluster{"X-array":dbl[], "Y-array":dbl[]})  [unwired: 7 in, 1 out]
      }
      n163 = call "2D to XY.vi"("error in (no error)"=w240, "X Array"=w241, "2D Z Array"=w242) -> ()  [unwired: 7 in, 2 out]
    }
    frame #8 {
      # "Utilities"
      n164 = call "X Units.vi"() -> ()  [unwired: 3 in, 1 out]
      n165 = call "DQ subVI.vi"() -> ()  [unwired: 11 in, 1 out]
      n166 = call "X Units.vi"() -> ()  [unwired: 3 in, 1 out]
      n167 = call "X Array Index to Range.vi"() -> ()  [unwired: 2 in, 1 out]
      n168 = call "X Array Range to Index.vi"() -> ()  [unwired: 2 in, 1 out]
      n169 = call "Hann Windows.vi"() -> ()  [unwired: 10 in, 2 out]
    }
  }
